vi "AMI MAG PHI IS.vi"(0 "Y-Axis Communications Config":T3, 1 "delta H (mT)":dbl=0.5, 2 "delta phi (deg)":dbl=0.5, 3 "sweep parameter":T1=enum."magnetic field", 4 "const phi?":bool, 5 "Z-Axis Communications Config":T3, 7 "target mag in (T)":dbl, 9 "target phi (deg)":dbl, 11 "error in (no error)":T2) -> (6 "target mag out (T)":dbl[](array[numeric]), 8 "phi array (deg)":dbl[](array[numeric]), 15 "error out":T2)   [LabVIEW 2013]
uses:
  measurement/measurement sweep parameter.ctl
  <vilib>/Analysis/1siggen.llb/Ramp Pattern by Delta.vi
  <vilib>/Analysis/NI_AALBase.lvlib
panel:
  out "current mag (kG)":dbl
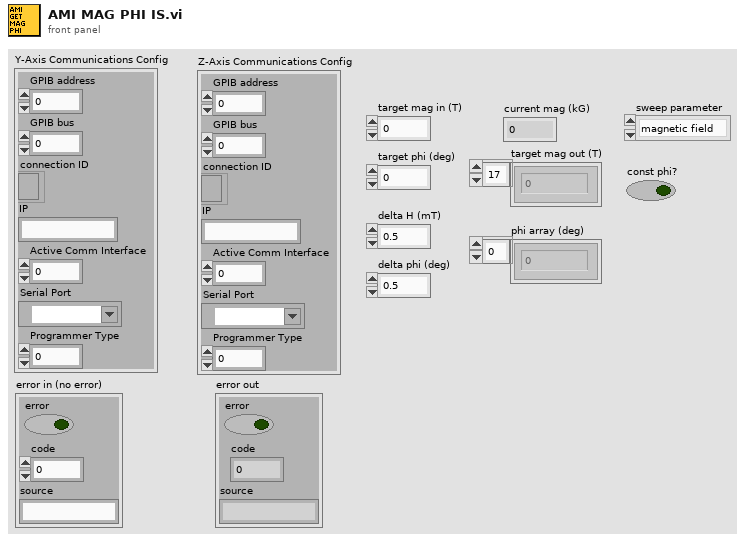
[diagram p1: front panel]
types:
  T1 = typedef "measurement sweep parameter.ctl" = enum16{"angle", "magnetic field"}
  T2 = cluster{"error":bool, "code":i32, "source":string}
  T3 = cluster{"GPIB address":i16, "GPIB bus":i16, "connection ID":refnum<k5>, "IP":string, "Active Comm Interface":u16, "Serial Port":refnum<visa-resource-name>, "Programmer Type":u16}
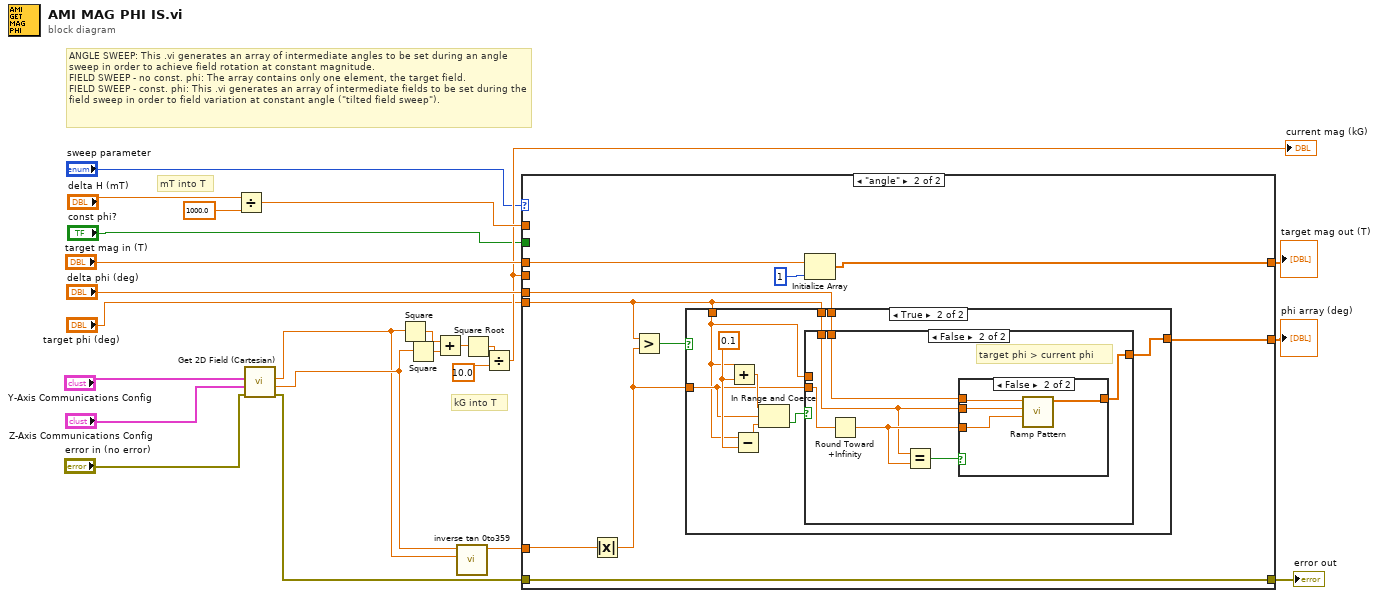
[diagram p0: block diagram]
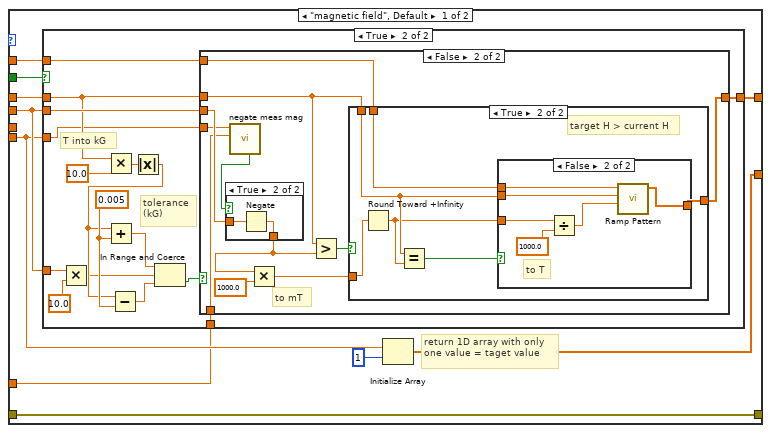
[diagram p2: hidden frame]
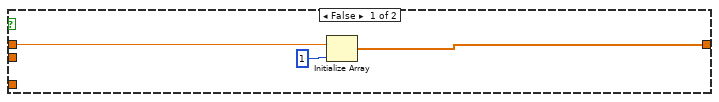
[diagram p3: hidden frame]
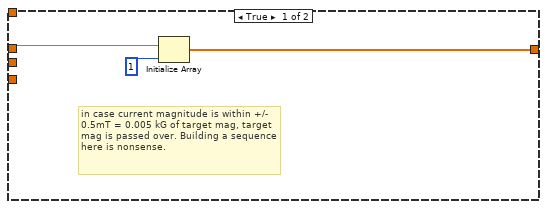
[diagram p4: hidden frame]
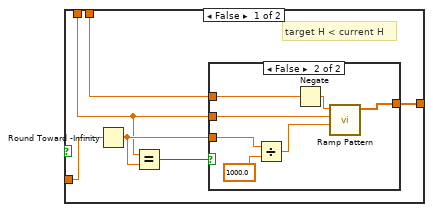
[diagram p6: hidden frame]
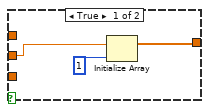
[diagram p7: hidden frame]
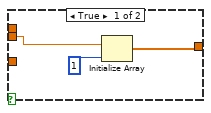
[diagram p8: hidden frame]
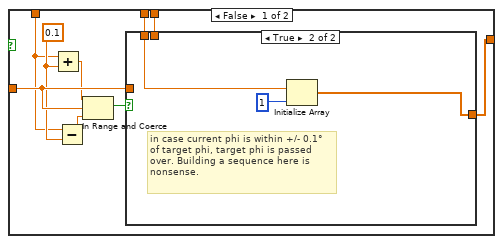
[diagram p9: hidden frame]
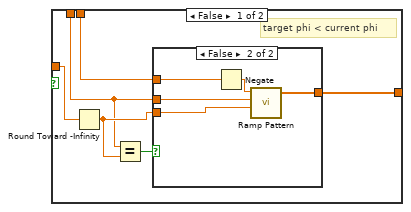
[diagram p10: hidden frame]
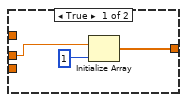
[diagram p11: hidden frame]
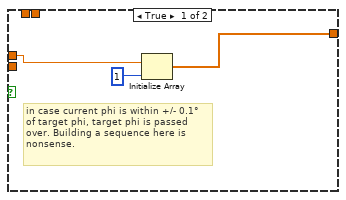
[diagram p12: hidden frame]
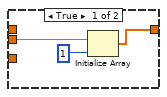
[diagram p13: hidden frame]
diagram:
  # "kG into T"
  # "mT into T"
  # "ANGLE SWEEP: This .vi generates an array of intermediate angles to be set during an angle sweep in order to achieve field rotation at constant magnitude.\nFIELD SWEEP - no const. phi: The array contains only one element, the target field.\nFIELD SWEEP - const. phi: This .vi generates an array of intermediate fields to be set during the field sweep in order to field variation at constant angle (\"tilted field sweep\")."
  n1 = Divide(x="delta H (mT)", y=1000.0) -> (x/y=w10:dbl)
  n2 = call <userlib>:"Get 2D Field (Cartesian).vi"("Y-Axis Communications Config"="Y-Axis Communications Config", "Z-Axis Communications Config"="Z-Axis Communications Config", "error in"="error in (no error)") -> ("Y-Axis Field (kG)"=w3:dbl, "Z-Axis Field (kG)"=w13:dbl, "error out"=w14:T2)  [unwired: 2 in, 1 out]
  n3 = Square(x=w3) -> (x^2=w20:dbl)
  n4 = Square(x=w13) -> (x^2=w19:dbl)
  n5 = Add(x=w20, y=w19) -> (x+y=w21:dbl)
  n6 = call "inverse tan 0to359.vi"("y coil"=w3, "z coil"=w13) -> ("phi (deg)"=w1:dbl)  [unwired: 9 in]
  n7 = Square Root(x=w21) -> (sqrt(x)=w6:dbl)
  n8 = Divide(x=w6, y=10.0) -> (x/y=w8:dbl)
  "current mag (kG)" <- w8
  n9 = case shown="\"angle\"" "sweep parameter" {
    tunnel: "target phi (deg)" -> [w26 w104]
    tunnel: w1 -> [w25 w102]
    tunnel: "delta phi (deg)" -> [_ w111]
    tunnel: [w32 w110] -> w17
    tunnel: [w30 w105] -> w12
    tunnel: "target mag in (T)" -> [w31 w106]
    tunnel: [w33 w109] -> w15
    tunnel: w14 -> [w33 w109]
    tunnel: "const phi?" -> [w29 _]
    tunnel: w8 -> [w27 _]
    tunnel: w10 -> [w28 _]
    frame "magnetic field", Default {
      # "return 1D array with only one value = taget value"
      n10 = case shown="True" w29 {
        tunnel: w31 -> [w36 w46]
        tunnel: [w35 w53] -> w30
        tunnel: w27 -> [_ w52]
        tunnel: w28 -> [_ w43]
        tunnel: w27 -> [_ w41]
        tunnel: w26 -> [_ w39]
        tunnel: w25 -> [_ w38]
        frame False {
          n11 = Initialize Array(w36, 1) -> (w35:dbl[])
        }
        frame True {
          w51 = 0.005
          # "tolerance (kG)"
          # "T into kG"
          n12 = Multiply(x=w41, y=10.0) -> (x*y=w40:dbl)
          n13 = Multiply(x=w46, y=10.0) -> (x*y=w45:dbl)
          n14 = Absolute Value(x=w45) -> (abs(x)=w44:dbl)
          n15 = Add(x=w44, y=w51) -> (x+y=w49:dbl)
          n16 = Subtract(x=w44, y=w51) -> (x-y=w50:dbl)
          n17 = In Range and Coerce(upper limit=w49, x=w40, lower limit=w50) -> (In Range?=w48:bool)  [unwired: 1 out]
          n18 = case shown="False" w48 {
            tunnel: w46 -> [w54 w60]
            tunnel: [w55 w63] -> w53
            tunnel: w52 -> [_ w62]
            tunnel: w43 -> [_ w64]
            tunnel: w39 -> [_ w58]
            tunnel: w38 -> [_ w57]
            frame True {
              # "in case current magnitude is within +/- 0.5mT = 0.005 kG of target mag, target mag is passed over. Building a sequence here is nonsense."
              n19 = Initialize Array(w54, 1) -> (w55:dbl[])
            }
            frame False {
              # "to mT"
              n20 = call "negate meas mag.vi"("current phi (deg)"=w57, "target phi (deg)"=w58) -> ("Negate measured mag?"=w59:bool)  [unwired: 9 in]
              n21 = case shown="True" w59 {
                tunnel: w62 -> [w68 w70]
                tunnel: [w68 w69] -> w61
                frame False {
                }
                frame True {
                  n22 = Negate(x=w70) -> (-x=w69:dbl)
                }
              }
              n23 = Multiply(x=w61, y=1000.0) -> (x*y=w66:dbl)
              n24 = Greater?(x=w60, y=w61) -> (0:w67:bool)
              n25 = case shown="True" w67 {
                tunnel: w60 -> [w71 w88]
                tunnel: w66 -> [w74 w90]
                tunnel: w64 -> [w76 w92]
                tunnel: [w75 w91] -> w63
                frame False {
                  # "target H < current H"
                  n26 = Round Toward -Infinity(1:w74) -> (0:w72:dbl)
                  n27 = Equal?(x=w71, y=w72) -> (x = y?=w73:bool)
                  n28 = case shown="False" w73 {
                    tunnel: w76 -> [_ w85]
                    tunnel: w71 -> [w77 w84]
                    tunnel: [w78 w83] -> w75
                    tunnel: w72 -> [_ w82]
                    frame True {
                      n29 = Initialize Array(w77, 1) -> (w78:dbl[])
                    }
                    frame False {
                      n30 = Divide(x=w82, y=1000.0) -> (x/y=w80:dbl)
                      n31 = Negate(x=w85) -> (-x=w86:dbl)
                      n32 = call-poly <vilib>:"Ramp Pattern.vi"("start"=w80, "end"=w84, "delta"=w86) -> ("Ramp Pattern"=w83:dbl[])  [unwired: 6 in, 2 out]
                    }
                  }
                }
                frame True {
                  # "target H > current H"
                  n33 = Round Toward +Infinity(x=w90) -> (ceil(x): smallest int >= x=w87:dbl)
                  n34 = Equal?(x=w88, y=w87) -> (x = y?=w89:bool)
                  n35 = case shown="False" w89 {
                    tunnel: w88 -> [w93 w101]
                    tunnel: w92 -> [_ w100]
                    tunnel: [w94 w99] -> w91
                    tunnel: w87 -> [_ w98]
                    frame True {
                      n36 = Initialize Array(w93, 1) -> (w94:dbl[])
                    }
                    frame False {
                      # "to T"
                      n37 = Divide(x=w98, y=1000.0) -> (x/y=w96:dbl)
                      n38 = call-poly <vilib>:"Ramp Pattern.vi"("start"=w96, "end"=w101, "delta"=w100) -> ("Ramp Pattern"=w99:dbl[])  [unwired: 6 in, 2 out]
                    }
                  }
                }
              }
            }
          }
        }
      }
      n39 = Initialize Array(w26, 1) -> (w32:dbl[])
    }
    frame "angle" {
      n40 = Absolute Value(x=w102) -> (abs(x)=w103:dbl)
      n41 = Greater?(x=w104, y=w103) -> (0:w108:bool)
      n42 = case shown="True" w108 {
        tunnel: w104 -> [w119 w146]
        tunnel: w103 -> [w116 w139]
        tunnel: w111 -> [w120 w145]
        tunnel: [w118 w144] -> w110
        tunnel: w104 -> [w112 w138]
        frame False {
          w113 = 0.1
          n43 = Add(x=w112, y=w113) -> (x+y=w115:dbl)
          n44 = Subtract(x=w112, y=w113) -> (x-y=w114:dbl)
          n45 = In Range and Coerce(upper limit=w115, x=w116, lower limit=w114) -> (In Range?=w117:bool)  [unwired: 1 out]
          n46 = case shown="True" w117 {
            tunnel: w116 -> [w124 _]
            tunnel: w120 -> [w125 _]
            tunnel: w119 -> [w121 w136]
            tunnel: [w126 w135] -> w118
            frame False {
              # "target phi < current phi"
              n47 = Round Toward -Infinity(1:w124) -> (0:w122:dbl)
              n48 = Equal?(x=w121, y=w122) -> (x = y?=w123:bool)
              n49 = case shown="False" w123 {
                tunnel: [w128 w133] -> w126
                tunnel: w125 -> [_ w132]
                tunnel: w122 -> [_ w130]
                tunnel: w121 -> [w127 w131]
                frame True {
                  n50 = Initialize Array(w127, 1) -> (w128:dbl[])
                }
                frame False {
                  n51 = Negate(x=w132) -> (-x=w134:dbl)
                  n52 = call-poly <vilib>:"Ramp Pattern.vi"("start"=w130, "end"=w131, "delta"=w134) -> ("Ramp Pattern"=w133:dbl[])  [unwired: 6 in, 2 out]
                }
              }
            }
            frame True {
              # "in case current phi is within +/- 0.1° of target phi, target phi is passed over. Building a sequence here is nonsense."
              n53 = Initialize Array(w136, 1) -> (w135:dbl[])
            }
          }
        }
        frame True {
          w141 = 0.1
          n54 = Add(x=w138, y=w141) -> (x+y=w143:dbl)
          n55 = Subtract(x=w138, y=w141) -> (x-y=w142:dbl)
          n56 = In Range and Coerce(upper limit=w143, x=w139, lower limit=w142) -> (In Range?=w140:bool)  [unwired: 1 out]
          n57 = case shown="False" w140 {
            tunnel: w146 -> [_ w151]
            tunnel: w139 -> [_ w150]
            tunnel: w145 -> [_ w155]
            tunnel: [w148 w154] -> w144
            tunnel: w138 -> [w147 _]
            frame True {
              # "in case current phi is within +/- 0.1° of target phi, target phi is passed over. Building a sequence here is nonsense."
              n58 = Initialize Array(w147, 1) -> (w148:dbl[])
            }
            frame False {
              # "target phi > current phi"
              n59 = Round Toward +Infinity(x=w150) -> (ceil(x): smallest int >= x=w152:dbl)
              n60 = Equal?(x=w151, y=w152) -> (x = y?=w153:bool)
              n61 = case shown="False" w153 {
                tunnel: w151 -> [w156 w162]
                tunnel: w155 -> [_ w161]
                tunnel: w152 -> [_ w160]
                tunnel: [w157 w159] -> w154
                frame True {
                  n62 = Initialize Array(w156, 1) -> (w157:dbl[])
                }
                frame False {
                  n63 = call-poly <vilib>:"Ramp Pattern.vi"("start"=w160, "end"=w162, "delta"=w161) -> ("Ramp Pattern"=w159:dbl[])  [unwired: 6 in, 2 out]
                }
              }
            }
          }
        }
      }
      n64 = Initialize Array(w106, 1) -> (w105:dbl[])
    }
  }
  "error out" <- w15
  "phi array (deg)" <- w17
  "target mag out (T)" <- w12
